vi "IdleCheck.vi"(8 "error in (no error)":errorcluster, 11 "S1.lvclass":refnum<class "S1.lvclass">) -> (0 "error out":errorcluster)   [LabVIEW 2018, in "S1.lvclass"]
uses:
  S1.lvclass
  S1.lvclass/S1.ctl
  Controller/GUI.lvclass
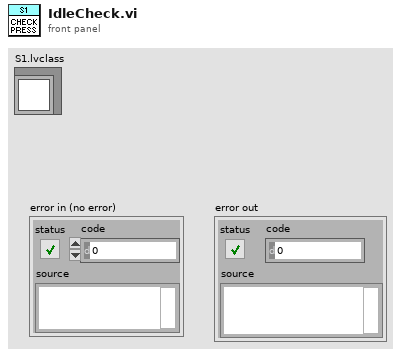
[diagram p1: front panel]
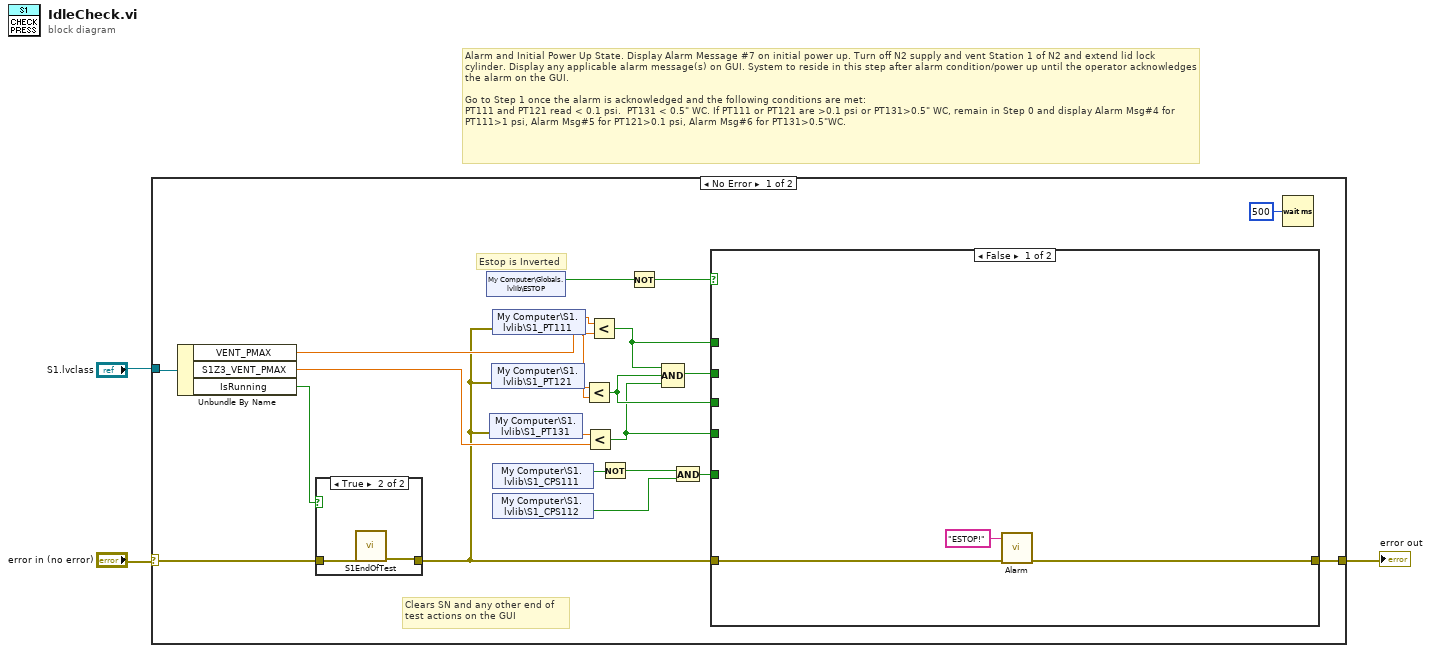
[diagram p0: block diagram]
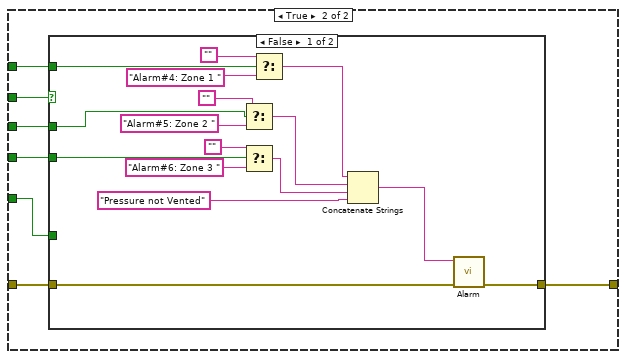
[diagram p3: hidden frame]
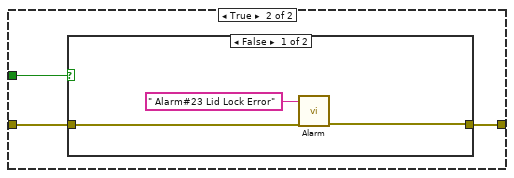
[diagram p4: hidden frame]
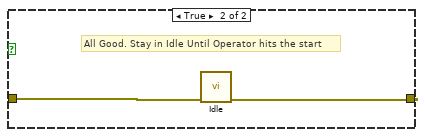
[diagram p5: hidden frame]
diagram:
  # "Alarm and Initial Power Up State. Display Alarm Message #7 on initial power up. Turn off N2 supply and vent Station 1 of N2 and extend lid lock cylinder. Display any applicable alarm message(s) on GUI. System to reside in this step after alarm condition/power up until the operator acknowledges the alarm on the GUI. \n\nGo to Step 1 once the alarm is acknowledged and the following conditions are met:\nPT111 and PT121 read < 0.1 psi.  PT131 < 0.5\" WC. If PT111 or PT121 are >0.1 psi or PT131>0.5\" WC, remain in Step 0 and display Alarm Msg#4 for PT111>1 psi, Alarm Msg#5 for PT121>0.1 psi, Alarm Msg#6 for PT131>0.5\"WC."
  n1 = case shown="No Error" "error in (no error)" {
    selector: "error in (no error)" -> [w5 w62]
    tunnel: [w15 w62] -> w2
    tunnel: "S1.lvclass" -> [w9 _]
    frame No Error {
      # "Clears SN and any other end of\ntest actions on the GUI"
      # "Estop is Inverted"
      n2 = Unbundle By Name(w9) -> ("VENT_PMAX"=w8:dbl, "S1Z3_VENT_PMAX"=w7:dbl, "IsRunning"=w6:bool)
      n3 = case shown="True" w6 {
        tunnel: w5 -> [w25 w27]
        tunnel: [w25 w26] -> w4
        frame False {
        }
        frame True {
          n4 = call "S1EndOfTest.vi"("error in"=w27) -> ("error out"=w26:errorcluster)  [unwired: 10 in]
        }
      }
      n5 = shared-variable "My Computer\\Globals.lvlib\\ESTOP"() -> (w17:bool)  [unwired: 1 in, 1 out]
      n6 = shared-variable "My Computer\\S1.lvlib\\S1_PT131"(error in=w4) -> (w18:dbl)  [unwired: 1 out]
      n7 = shared-variable "My Computer\\S1.lvlib\\S1_PT121"(error in=w4) -> (w23:dbl)  [unwired: 1 out]
      n8 = shared-variable "My Computer\\S1.lvlib\\S1_PT111"(error in=w4) -> (w24:dbl)  [unwired: 1 out]
      n9 = shared-variable "My Computer\\S1.lvlib\\S1_CPS111"() -> (w13:bool)  [unwired: 1 in, 1 out]
      n10 = shared-variable "My Computer\\S1.lvlib\\S1_CPS112"() -> (w12:bool)  [unwired: 1 in, 1 out]
      n11 = Less?(x=w23, y=w8) -> (x < y?=w20:bool)
      n12 = Less?(x=w18, y=w7) -> (x < y?=w19:bool)
      n13 = Less?(x=w24, y=w8) -> (x < y?=w21:bool)
      n14 = Not(x=w13) -> (.not. x?=w14:bool)
      n15 = Not(x=w17) -> (.not. x?=w16:bool)
      n16 = Compound Arithmetic op=AND(w21, w20, w19) -> (w22:bool)
      n17 = And(x=w14, y=w12) -> (x .and. y?=w11:bool)
      n18 = case shown="False" w16 {
        tunnel: w22 -> [_ w37]
        tunnel: w21 -> [_ w35]
        tunnel: w20 -> [_ w34]
        tunnel: w19 -> [_ w33]
        tunnel: w4 -> [w30 w32]
        tunnel: [w29 w36] -> w15
        tunnel: w11 -> [_ w31]
        frame False {
          n19 = call "Alarm.vi"("error in"=w30, "Alarm"="ESTOP!" ("Status")) -> ("error out"=w29:errorcluster)  [unwired: 9 in]
        }
        frame True {
          n20 = case shown="False" w37 {
            tunnel: w32 -> [w53 w56]
            tunnel: [w40 w55] -> w36
            tunnel: w35 -> [w51 _]
            tunnel: w34 -> [w47 _]
            tunnel: w33 -> [w45 _]
            tunnel: w31 -> [_ w54]
            frame False {
              n21 = Select(t="", s=w47, f="Alarm#5: Zone 2 " ("Status")) -> (s? t:f=w42:string)
              n22 = Select(t="", s=w45, f="Alarm#6: Zone 3 " ("Status")) -> (s? t:f=w41:string)
              n23 = Select(t="", s=w51, f="Alarm#4: Zone 1 " ("Status")) -> (s? t:f=w43:string)
              n24 = Concatenate Strings(w43, w42, w41, "Pressure not Vented" ("Status")) -> (w38:string)
              n25 = call "Alarm.vi"("error in"=w53, "Alarm"=w38) -> ("error out"=w40:errorcluster)  [unwired: 9 in]
            }
            frame True {
              n26 = case shown="False" w54 {
                tunnel: w56 -> [w59 w61]
                tunnel: [w58 w60] -> w55
                frame False {
                  n27 = call "Alarm.vi"("error in"=w59, "Alarm"=" Alarm#23 Lid Lock Error" ("Status")) -> ("error out"=w58:errorcluster)  [unwired: 9 in]
                }
                frame True {
                  # "All Good. Stay in Idle Until Operator hits the start"
                  n28 = call "Idle.vi"("error in"=w61) -> ("error out"=w60:errorcluster)  [unwired: 10 in]
                }
              }
            }
          }
        }
      }
      n29 = Wait (ms)(milliseconds to wait=u32 500) -> ()  [unwired: 1 out]
    }
    frame Error {
    }
  }
  "error out" <- w2
